vi "Main.vi"() -> ()   [LabVIEW 2020]
doc: "This template is for the Queued Message Handler design pattern.\n\nThe Event Handling Loop generates messages based on user interface actions.\n\nThe Message Handling Loop processes messages generated by the Event Handling Loop, or by other messages. The messages are string values, so new messages can be added easily to the Message Cases case structure in the Message Handling Loop. Each message cluster can also provide an optional value for Message Data, which is a variant that can be converted to whatever message-specific data is required."
uses:
  controls/Search button.ctl
  Panther Dashboard Library/Module type--enum.ctl
  controls/UI Data.ctl
  Panther Dashboard Library/DQMH Modules Info--cluster.ctl
  Panther Dashboard Library/Documentation--cluster.ctl
  support/User Event - Stop/User Events Refs--cluster.ctl
  Panther Dashboard Library/Project Name and Ref--cluster.ctl
  Panther Dashboard Library/Maps List and refs--cluster.ctl
  <vilib>/National Instruments/Tree Map/Tree Map Data.ctl
  <vilib>/Utility/miscctls.llb/LVPointTypeDef.ctl
  support/Message Queue/Enqueue Message (Array).vi
  support/Message Queue/Enqueue Message (Single).vi
  <vilib>/National Instruments/Tree Map/API/List Roots.vi
  <vilib>/National Instruments/Tree Map/Utility/Into Tree Control Items.vi
  <vilib>/Utility/error.llb/Error Cluster From Error Code.vi
  <vilib>/ErrorRing/Error Ring.xnode
  support/Message Queue/Message Queue.lvlib
  support/User Event - Stop/User Events.lvlib
  <vilib>/National Instruments/Tree Map/Tree Map.lvlib
  Panther Dashboard Library/Panther Dashboard.lvlib
  PantherSniffer/Source/Libraries/MQTT_Client/MQTT_Client.lvlib
panel:
  in  "Include Dependencies":bool
  in  "Projects":string(combo)
  in  "Refresh":T1
  in  "DQMH List":string(tree) caption="Tree 2"
  out "Event Connector Pane":picture
  in  "Open Event FP":bool
  in  "Module ID":i32 caption="Numeric" format="Module ID : %d"
  in  "Show Diagram":bool
  in  "Hide Panel":bool
  in  "Show Panel":bool
  in  "Stop Instance":bool
  in  "Stop Module":bool
  out "Running?":bool
  out "Module type":T2
  in  "Open API Tester":bool
  out "Module Description":string
  out "Event Description":string
  out "Messages":string
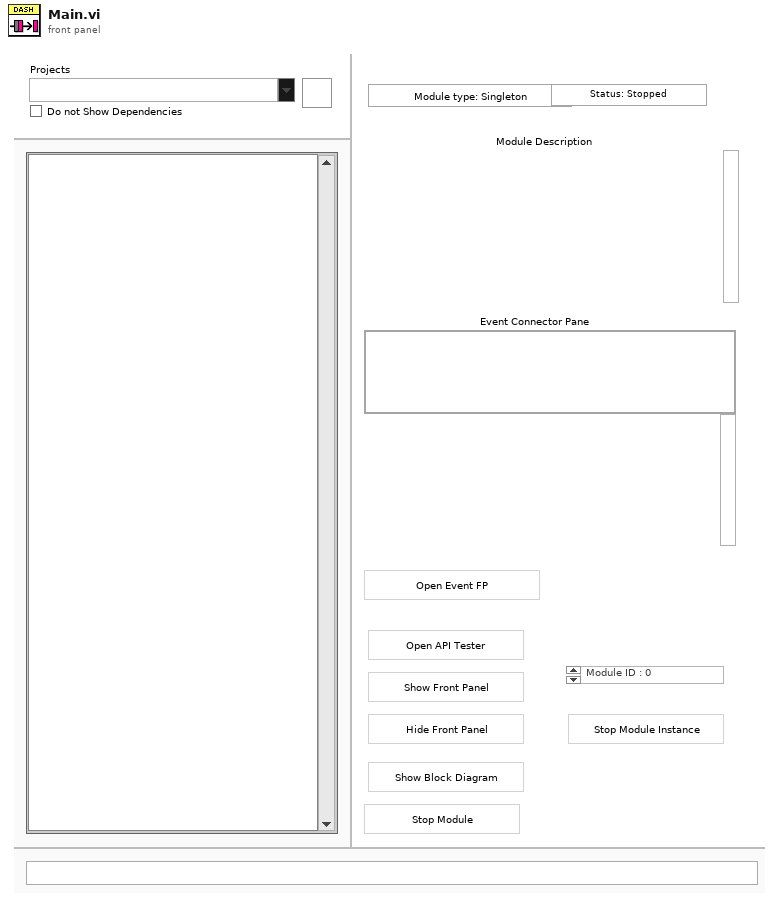
[diagram p1: front panel]
types:
  T1 = typedef "Search button.ctl" = bool
  T2 = typedef "Panther Dashboard.lvlib/Module type--enum.ctl" = enum16{"Module type: Singleton", "Module type: Cloneable"}
  T3 = typedef "UI Data.ctl" = cluster{"DQMH Modules Info":T4, "Documentation":T5, "FP Ctrs Refs":cluster{"Open API Tester":refnum<vi>, "Run Request VI":refnum<vi>, "Show Diagram":refnum<vi>, "Hide Panel":refnum<vi>, "Show Panel":refnum<vi>, "Stop All":refnum<vi>, "Stop Module":refnum<vi>}, "User Events":T6, "Project":T7, "UI Elements":cluster{"Connector pane img":picture, "Module selected type":T2, "DQMH Module Name":string, "Module ID":i32}, "DQMH Refs":cluster{"Event vi Ref":refnum<vi>, "DQMH Module Selected Ref":refnum<vi>}, "Maps":T8, "Tree Control Ref":refnum<vi>}
  T4 = typedef "Panther Dashboard.lvlib/DQMH Modules Info--cluster.ctl" = cluster{"DQMH Modules Refs":refnum<vi>[], "Modules List":string[], "Modules Descriptions":string[], "Modules Paths":path[], "Modules type":T2[]}
  T5 = typedef "Panther Dashboard.lvlib/Documentation--cluster.ctl" = cluster{"Module Description":string, "Event Description":string}
  T6 = typedef "User Events.lvlib/User Events Refs--cluster.ctl" = cluster{"Stop Event":refnum<user-event>, "Message event ":refnum<user-event>, "DQMH Mod Ref":refnum<user-event>}
  T7 = typedef "Panther Dashboard.lvlib/Project Name and Ref--cluster.ctl" = cluster{"Project Ref":refnum<vi>, "Project Name Selection":string, "Include Dependencies":bool}
  T8 = typedef "Panther Dashboard.lvlib/Maps List and refs--cluster.ctl" = cluster{"Tree Map":T9, "References Map":map{string, refnum<vi>}}
  T9 = typedef "Tree Map.lvlib/Tree Map Data.ctl" = map{string, cluster{"Child Paths Set":set{string}, "Name":string, "Data":string, "Attributes":map{string, string}}}
  T10 = typedef "Message Queue.lvlib/All Message Queues.ctl" = cluster{"UI":refnum<queue>}
  T11 = typedef "LVPointTypeDef.ctl" = cluster{"Horizontal":i16, "Vertical":i16}
  T12 = enum8{"Enabled", "Disabled", "Disabled and Grayed Out"}
  T13 = enum32{"Invalid", "Standard", "Closed", "Hidden", "Minimized", "Maximized"}
  T14 = cluster{"Open API Tester":refnum<vi>, "Open Event FP":refnum<vi>, "Show Diagram":refnum<vi>, "Hide Panel":refnum<vi>, "Show Panel":refnum<vi>, "Stop Instance":refnum<vi>, "Stop Module":refnum<vi>}
  T15 = cluster{"Left Cell String":string, "Child Text":string[], "Child Tag":string, "Item Indent":i32, "Child Only?":bool, "Glyph Index":i32}[]
  T16 = cluster{"Open API Tester":refnum<vi>, "Run Request VI":refnum<vi>, "Show Diagram":refnum<vi>, "Hide Panel":refnum<vi>, "Show Panel":refnum<vi>, "Stop All":refnum<vi>, "Stop Module":refnum<vi>}
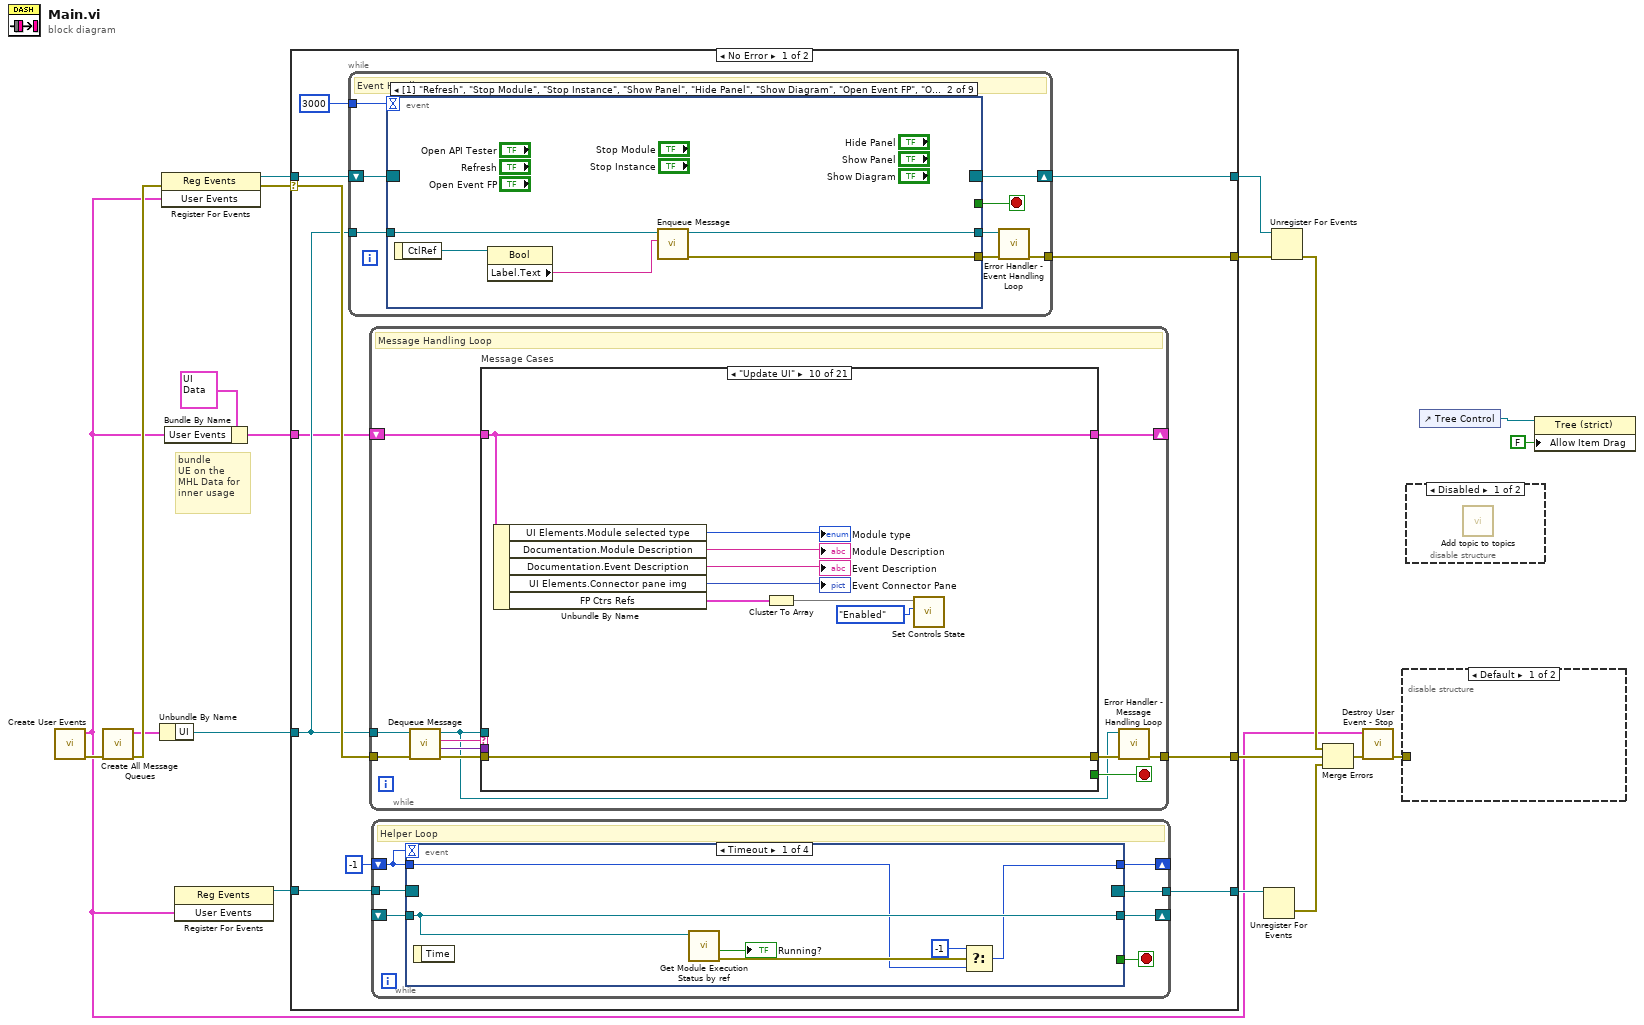
[diagram p0: block diagram]
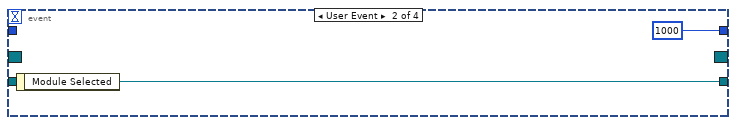
[diagram p3: hidden frame]
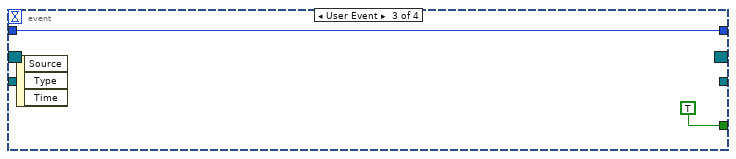
[diagram p4: hidden frame]
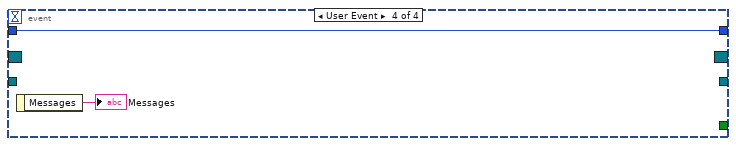
[diagram p5: hidden frame]
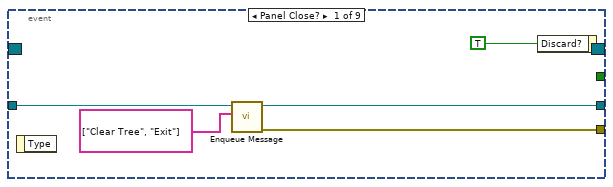
[diagram p6: hidden frame]
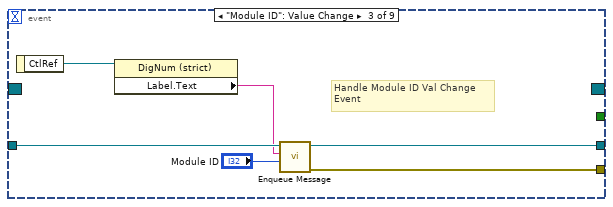
[diagram p7: hidden frame]
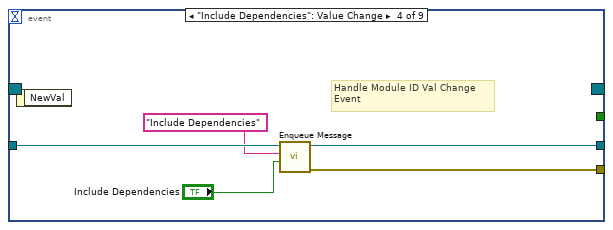
[diagram p8: hidden frame]
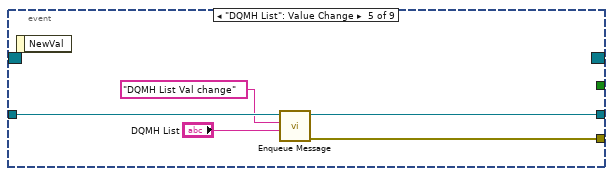
[diagram p9: hidden frame]
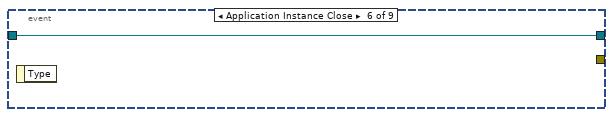
[diagram p10: hidden frame]
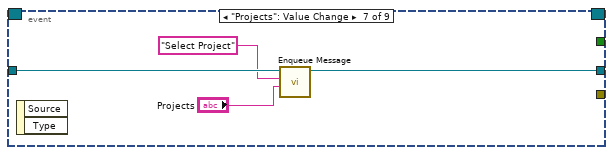
[diagram p11: hidden frame]
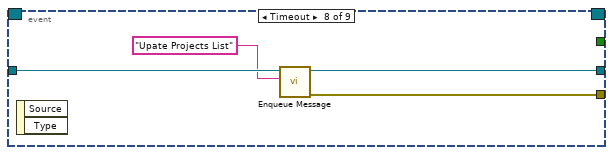
[diagram p12: hidden frame]
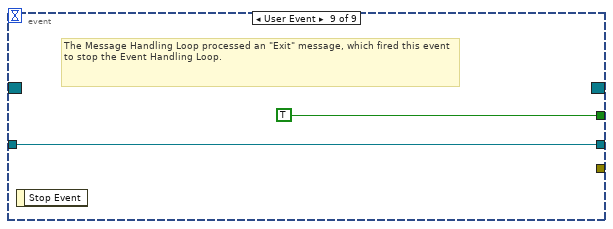
[diagram p13: hidden frame]
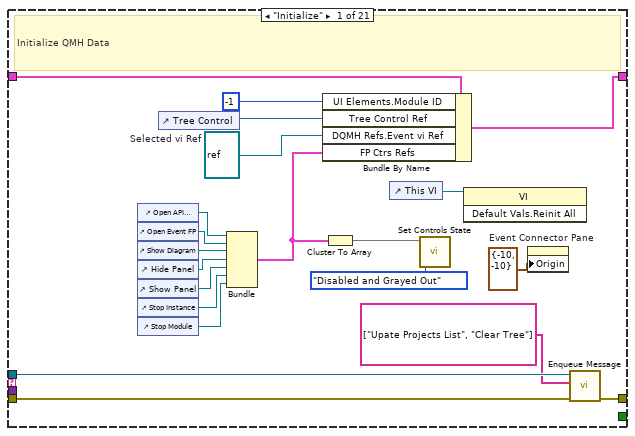
[diagram p14: hidden frame]
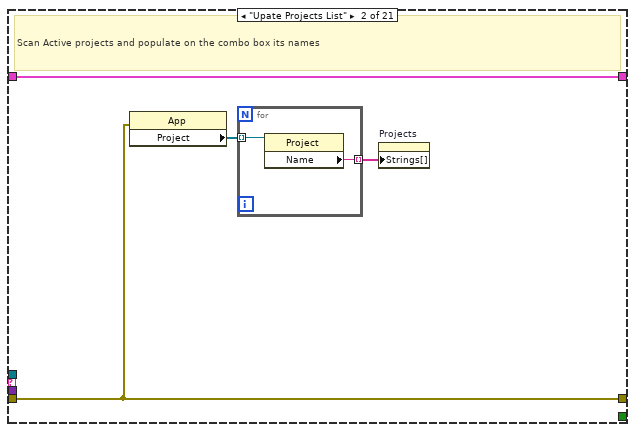
[diagram p15: hidden frame]
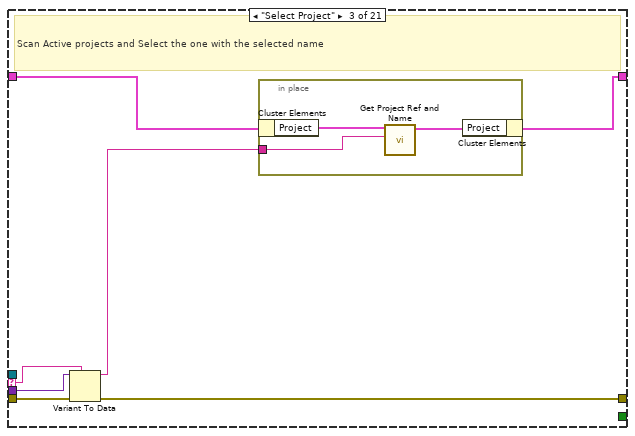
[diagram p16: hidden frame]
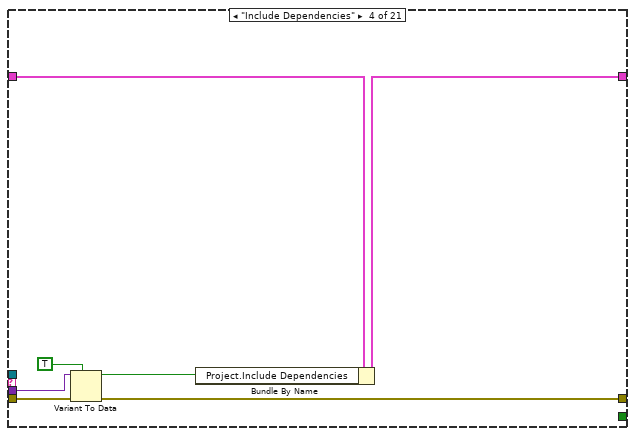
[diagram p17: hidden frame]
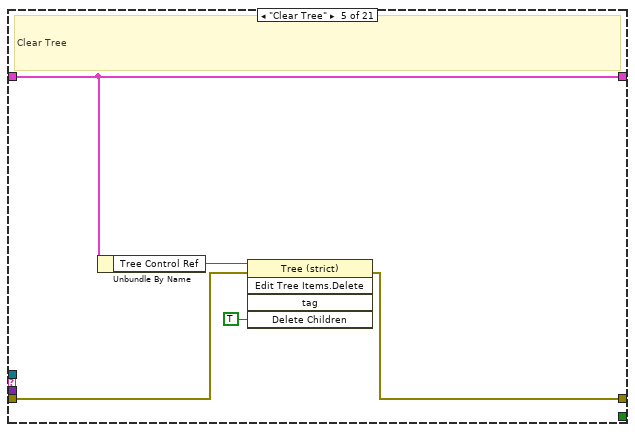
[diagram p18: hidden frame]
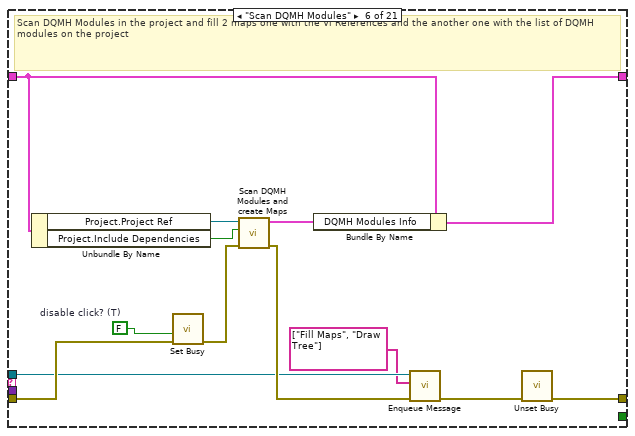
[diagram p19: hidden frame]
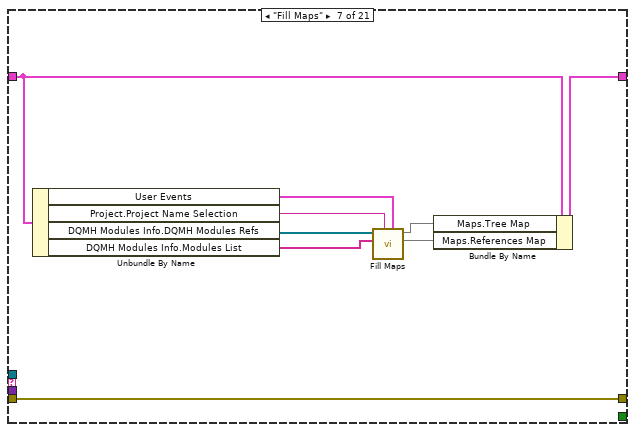
[diagram p20: hidden frame]
diagram:
  # "bundle\nUE on the\nMHL Data for\ninner usage"
  n1 = call "Create User Events.vi"() -> ("error out"=w19:errorcluster, "User Events"=w3:T6)  [unwired: 10 in]
  n2 = call "Create All Message Queues.vi"("error in (no error)"=w19) -> ("error out"=w13:errorcluster, "Message Queues out"=w11:T10)  [unwired: 9 in]
  n3 = Unbundle By Name(w11) -> ("UI"=w10:refnum<queue>)
  n4 = register-events(error in=w13, w3) -> (reference out=w7:refnum<event-registration>, error out=w12:errorcluster)  [unwired: 1 in]
  n5 = Bundle By Name(cluster=T3 {"DQMH Modules Info"={"DQMH Modules Refs"=[], "Modules List"=[], "Modules Descriptions"=[], "Modules Paths"=[], "Modules type"=[]}, "Documentation"={"Module Description"="", "Event Description"=""}, "FP Ctrs Refs"={"Open API Tester"=refnum, "Run Request VI"=refnum, "Show Diagram"=refnum, "Hide Panel"=refnum, "Show Panel"=refnum, "Stop All"=refnum, "Stop Module"=refnum}, "User Events"={"Stop Event"=refnum, "Message event "=refnum, "DQMH Mod Ref"=refnum}, "Project"={"Project Ref"=refnum, "Project Name Selection"="", "Include Dependencies"=FALSE}, "UI Elements"={"Connector pane img"=bytes[0], "Module selected type"=enum."Module type: Singleton", "DQMH Module Name"="", "Module ID"=0}, "DQMH Refs"={"Event vi Ref"=refnum, "DQMH Module Selected Ref"=refnum}, "Maps"={"Tree Map"={}, "References Map"={}}, "Tree Control Ref"=refnum} ("Data Cluster"), "User Events"=w3) -> (w6:T3)
  n6 = register-events(w3) -> (reference out=w5:refnum<event-registration>)  [unwired: 2 in, 1 out]
  n7 = case shown="No Error" w12 {
    selector: w12 -> [w29 w288]
    tunnel: [w31 _] -> w20
    tunnel: [w30 w288] -> w15
    tunnel: w10 -> [w28 _]
    tunnel: [w27 w287] -> w9
    tunnel: w7 -> [w26 w287]
    tunnel: w6 -> [w25 _]
    tunnel: w5 -> [w24 w286]
    tunnel: [w23 w286] -> w4
    frame No Error {
      n8 = while {
        tunnel: w28 -> [w56]
        shift-right: [w54] -> w27
        shift-left: w26 -> [w55]
        tunnel: [w57] -> w30
        tunnel: 3000 -> [w51]
        stop <- w53 stop-if-true
        # "Event Handling Loop"
        n9 = event shown="[1] \"Refresh\", \"Stop Module\", \"Stop Instance\", \"Show Panel\", \"Hide Panel\", \"Show Diagram\", \"Open Event FP\", \"Open API Tester\": Value Change" {
          selector: w55 -> [_ _ _ _ _ _ _ _ _]
          dyn-events: [_ _ _ _ _ _ _ _ _] -> w54
          timeout: w51 -> [_ _ _ _ _ _ _ _ _]
          tunnel: [_ _ _ _ _ _ _ _ TRUE ("Discard?")] -> w53
          tunnel: w56 -> [w61 w67 w73 w78 w84 w85 w89 w93 w95]
          tunnel: [w63 w68 w74 w79 w80 _ _ w90 _] -> w58
          tunnel: [w60 w65 w71 w77 w83 w85 w88 w92 w95] -> w52
          event Panel Close? {
            n10 = event-data() -> ()  [unwired: 1 in, 1 out]
            n11 = call-poly "Enqueue Message.vi"("Message Array"=string[] ["Clear Tree", "Exit"] ("Message"), "Message Queue"=w61) -> ("error out"=w63:errorcluster, "dup Message Queue"=w60:refnum<queue>)  [unwired: 8 in]
            n12 = event-data("Discard?"=TRUE) -> ()  [unwired: 1 in, 1 out]
          }
          event "Stop Module", "Stop Instance", "Show Panel", "Hide Panel", "Show Diagram", "Open Event FP", "Open API Tester": Value Change {
            n13 = event-data() -> ("CtlRef"=w66:refnum<vi>)  [unwired: 1 in]
            n14 = property class="Bool"(reference=w66) -> ("Label.Text"=w64:string)  [unwired: 1 in, 2 out]
            n15 = call-poly "Enqueue Message.vi"("Message"=w64, "Message Queue"=w67) -> ("error out"=w68:errorcluster, "dup Message Queue"=w65:refnum<queue>)  [unwired: 8 in]
          }
          event "Module ID": Value Change {
            # "Handle Module ID Val Change\nEvent"
            n16 = event-data() -> ("CtlRef"=w72:refnum<vi>)  [unwired: 1 in]
            n17 = property class="DigNum (strict)"(reference=w72) -> ("Label.Text"=w70:string)  [unwired: 1 in, 2 out]
            n18 = call-poly "Enqueue Message.vi"("Message Data"="Module ID", "Message"=w70, "Message Queue"=w73) -> ("error out"=w74:errorcluster, "dup Message Queue"=w71:refnum<queue>)  [unwired: 7 in]
          }
          event "Include Dependencies": Value Change {
            # "Handle Module ID Val Change\nEvent"
            n19 = event-data() -> ()  [unwired: 1 in, 1 out]
            n20 = call-poly "Enqueue Message.vi"("Message Data"="Include Dependencies", "Message"="Include Dependencies", "Message Queue"=w78) -> ("error out"=w79:errorcluster, "dup Message Queue"=w77:refnum<queue>)  [unwired: 7 in]
          }
          event "DQMH List": Value Change {
            n21 = event-data() -> ()  [unwired: 1 in, 1 out]
            n22 = call-poly "Enqueue Message.vi"("Message Data"="DQMH List", "Message"="DQMH List Val change", "Message Queue"=w84) -> ("error out"=w80:errorcluster, "dup Message Queue"=w83:refnum<queue>)  [unwired: 7 in]
          }
          event Application Instance Close {
            n23 = event-data() -> ()  [unwired: 1 in, 1 out]
          }
          event "Projects": Value Change {
            n24 = event-data() -> ()  [unwired: 1 in, 2 out]
            n25 = call-poly "Enqueue Message.vi"("Message Data"="Projects", "Message"="Select Project", "Message Queue"=w89) -> ("dup Message Queue"=w88:refnum<queue>)  [unwired: 7 in, 1 out]
          }
          event Timeout {
            n26 = event-data() -> ()  [unwired: 1 in, 2 out]
            n27 = call-poly "Enqueue Message.vi"("Message"="Upate Projects List", "Message Queue"=w93) -> ("error out"=w90:errorcluster, "dup Message Queue"=w92:refnum<queue>)  [unwired: 8 in]
          }
          event User Event {
            # "The Message Handling Loop processed an \"Exit\" message, which fired this event to stop the Event Handling Loop."
            n28 = event-data() -> ()  [unwired: 1 in, 1 out]
          }
        }
        n29 = call "Error Handler - Event Handling Loop.vi"("error in (no error)"=w58, "Message Queue"=w52) -> ("dup error in"=w57:errorcluster)  [unwired: 8 in, 1 out]
      }
      n30 = while {
        tunnel: w28 -> [w97]
        shift-right: [w101] -> _
        shift-left: w25 -> [w102]
        tunnel: w29 -> [w106]
        tunnel: [w104] -> w31
        stop <- w100 stop-if-true
        # "Message Handling Loop"
        n31 = call "Dequeue Message.vi"("error in (no error)"=w106, "Message Queue"=w97) -> ("error out"=w105:errorcluster, "Message Data"=w98:variant, "Message"=w99:string, "dup Message Queue"=w96:refnum<queue>)  [unwired: 6 in]
        n32 = case "Message Cases" shown="\"Update UI\"" w99 {
          selector: w99 -> [_ _ w137 _ _ _ _ _ _ _ _ w217 _ _ _ _ _ _ _ _ w276]
          tunnel: w96 -> [w123 _ _ _ _ w161 _ _ w192 _ _ _ _ w231 _ _ _ _ _ w269 _]
          tunnel: w105 -> [w127 w128 w140 w150 w155 w167 w177 w184 w203 w212 _ w223 w229 w235 w240 w246 w253 w260 w263 w272 _]
          tunnel: [w126 w128 w139 w148 w154 w164 w177 w183 w201 w212 w213 w222 w228 w234 w239 w245 w252 w256 w262 w274 w278] -> w103
          tunnel: w102 -> [w125 w131 w136 w149 w152 w160 w176 w181 w198 w211 w216 w220 w225 w233 w237 w244 w251 w255 w261 w266 w277]
          tunnel: [w124 w131 w134 w145 w152 w163 w172 w181 w196 w211 w216 w220 w225 w233 w237 w244 w248 w255 w261 w266 w277] -> w101
          tunnel: [_ _ _ _ _ _ _ _ _ _ _ _ _ _ _ _ _ _ _ TRUE _] -> w100
          tunnel: w98 -> [_ _ w138 w147 _ _ _ _ w200 _ _ _ _ _ _ _ w250 w254 _ w267 _]
          frame "Initialize" {
            w107 = refnum<vi> refnum  # Selected vi Ref
            # "Initialize QMH Data"
            n33 = control-ref of="Open API Tester"() -> (w115:refnum<vi>)
            n34 = control-ref of="Open Event FP"() -> (w116:refnum<vi>)
            n35 = control-ref of="Show Diagram"() -> (w117:refnum<vi>)
            n36 = control-ref of="Hide Panel"() -> (w118:refnum<vi>)
            n37 = control-ref of="Show Panel"() -> (w119:refnum<vi>)
            n38 = control-ref of="Stop Instance"() -> (w120:refnum<vi>)
            n39 = control-ref of="Stop Module"() -> (w121:refnum<vi>)
            n40 = control-ref of="Tree Control"() -> (w108:refnum<vi>)
            n41 = Bundle("Open API Tester"=w115, "Open Event FP"=w116, "Show Diagram"=w117, "Hide Panel"=w118, "Show Panel"=w119, "Stop Instance"=w120, "Stop Module"=w121) -> (w110:T14)  [unwired: 1 in]
            n42 = Bundle By Name(cluster=w125, "UI Elements.Module ID"=-1 ("Module ID"), "Tree Control Ref"=w108, "DQMH Refs.Event vi Ref"=w107, "FP Ctrs Refs"=w110) -> (w124:T3)
            n43 = Cluster To Array(cluster=w110) -> (array=w114:refnum<vi>[])
            n44 = control-ref of="This VI"() -> (w112:refnum<vi>)
            n45 = call "Set Controls State.vi"("Disabled"=T12."Disabled and Grayed Out", "Ctrl Refs"=w114) -> ()  [unwired: 10 in]
            n46 = invoke class="VI" method="Default Vals.Reinit All"(reference=w112) -> ()  [unwired: 2 in, 3 out]
            n47 = property on="Event Connector Pane" class="Pict"("Origin"=T11 {"Horizontal"=-10, "Vertical"=-10}) -> ()  [unwired: 2 in, 2 out]
            n48 = call-poly "Enqueue Message.vi"("error in (no error)"=w127, "Message Array"=string[] ["Upate Projects List", "Clear Tree"] ("Initial Step"), "Message Queue"=w123) -> ("error out"=w126:errorcluster)  [unwired: 7 in, 1 out]
          }
          frame "Upate Projects List" {
            # "Scan Active projects and populate on the combo box its names"
            n49 = property class="App"(error in=w128) -> ("Project"=w130:refnum<vi>[])  [unwired: 1 in, 2 out]
            n50 = for {
              tunnel: w130 -> [w133] mode=indexing
              tunnel: [w132] -> w129 mode=indexing
              n51 = property class="Project"(reference=w133) -> ("Name"=w132:string)  [unwired: 1 in, 2 out]
            }
            n52 = property on="Projects" class="CmbBox"("Strings[]"=w129) -> ()  [unwired: 2 in, 2 out]
          }
          frame "Select Project" {
            # "Scan Active projects and Select the one with the selected name"
            n53 = Variant To Data(error in=w140, type=w137, Variant=w138) -> (data=w135:string, error out=w139:errorcluster)
            n54 = in-place {
              in-place-border: w135 -> [w143]
              n55 = in-place-cluster #1(w136) -> ("Project"=w141:T7)
              n56 = call "Get Project Ref and Name.vi"("Project Name Selection"=w143, "ProjectIn"=w141) -> ("Project out"=w142:T7)  [unwired: 9 in]
              n57 = in-place-cluster #1("Project"=w142) -> (w134:T3)
            }
          }
          frame "Include Dependencies" {
            n58 = Variant To Data(error in=w150, type=TRUE, Variant=w147) -> (data=w144:bool, error out=w148:errorcluster)
            n59 = Bundle By Name(cluster=w149, "Project.Include Dependencies"=w144) -> (w145:T3)
          }
          frame "Clear Tree" {
            # "Clear Tree"
            n60 = Unbundle By Name(w152) -> ("Tree Control Ref"=w151:refnum<vi>)
            n61 = invoke on="Invoke Node" class="Tree (strict)" method="Edit Tree Items.Delete"(reference=w151, error in=w155, "Delete Children"=TRUE ("Delete Children?")) -> (error out=w154:errorcluster)  [unwired: 2 in, 4 out]
          }
          frame "Scan DQMH Modules" {
            w158 = FALSE  # disable click? (T)
            # "Scan DQMH Modules in the project and fill 2 maps one with the Vi References and the another one with the list of DQMH modules on the project"
            n62 = Unbundle By Name(w160) -> ("Project.Project Ref"=w159:refnum<vi>, "Project.Include Dependencies"=w156:bool)
            n63 = call <vilib>:"Set Busy.vi"("error in (no error)"=w167, "disable click? (T)"=w158) -> ("error out"=w166:errorcluster)  [unwired: 8 in, 1 out]
            n64 = call "Scan DQMH Modules and create Maps.vi"("error in"=w166, "Include Dependencies"=w156, "Project"=w159) -> ("error out"=w168:errorcluster, "DQMH Modules Info"=w162:T4)  [unwired: 7 in]
            n65 = Bundle By Name(cluster=w160, "DQMH Modules Info"=w162) -> (w163:T3)
            n66 = call-poly "Enqueue Message.vi"("error in (no error)"=w168, "Message Array"=string[] ["Fill Maps", "Draw Tree"] ("Message"), "Message Queue"=w161) -> ("error out"=w165:errorcluster)  [unwired: 7 in, 1 out]
            n67 = call <vilib>:"Unset Busy.vi"("error in (no error)"=w165) -> ("error out"=w164:errorcluster)  [unwired: 10 in]
          }
          frame "Fill Maps" {
            n68 = Unbundle By Name(w176) -> ("User Events"=w169:T6, "Project.Project Name Selection"=w173:string, "DQMH Modules Info.DQMH Modules Refs"=w175:refnum<vi>[], "DQMH Modules Info.Modules List"=w174:string[])
            n69 = call "Fill Maps.vi"("User Events"=w169, "Project Selected"=w173, "Module names"=w174, "DQMH Modules"=w175) -> ("map ref out"=w170:map{string, refnum<vi>}, "Tree Map out"=w171:T9)  [unwired: 5 in, 1 out]
            n70 = Bundle By Name(cluster=w176, "Maps.Tree Map"=w171, "Maps.References Map"=w170) -> (w172:T3)
          }
          frame "Draw Tree" {
            # "Draw  DQMH List with all the DQMH Modules listed, first we need to clean the tree list"
            n71 = Unbundle By Name(w181) -> ("Tree Control Ref"=w178:refnum<vi>, "Maps.Tree Map"=w180:T9)
            n72 = call <vilib>:"Tree Map to Tree Control Items.vi"("Tree Map In"=w180) -> ("Tree Control Items"=w179:T15)  [unwired: 10 in]
            n73 = call "Draw Tree.vi"("Tree Control Items"=w179, "TreeControl in"=w178) -> ("error out"=w182:errorcluster)  [unwired: 9 in]
            n74 = Merge Errors(w182, w184) -> (w183:errorcluster)
          }
          frame "DQMH List Val change" {
            # "DQMH List has a value change"
            n75 = Unbundle By Name(w198) -> ("Maps.Tree Map"=w197:T9, "Maps.References Map"=w194:map{string, refnum<vi>}, "DQMH Modules Info"=w193:T4)
            n76 = Variant To Data(error in=w203, type="" ("DQMH List"), Variant=w200) -> (data=w195:string, error out=w202:errorcluster)
            n77 = call "Get List Information.vi"("List Selection"=w195, "DQMH Modules Info"=w193, "References Map"=w194, "Tree Map"=w197) -> ("Documentation"=w190:T5, "Module Type"=w188:T2, "Vi out"=w187:refnum<vi>, "Library name"=w186:string, "VI Connector Pane"=w189:picture, "DQMH Lib"=w185:refnum<vi>)  [unwired: 2 in]
            n78 = Bundle By Name(cluster=w198, "DQMH Refs.DQMH Module Selected Ref"=w185, "UI Elements.DQMH Module Name"=w186, "DQMH Refs.Event vi Ref"=w187, "UI Elements.Module selected type"=w188, "Documentation"=w190, "UI Elements.Connector pane img"=w189) -> (w196:T3)
            n79 = call-poly "Enqueue Message.vi"("error in (no error)"=w202, "Message Array"=string[] ["Get Module Status", "Update UI"] ("Message"), "Message Queue"=w192) -> ("error out"=w201:errorcluster)  [unwired: 7 in, 1 out]
          }
          frame "Update UI" {
            n80 = Unbundle By Name(w211) -> ("UI Elements.Module selected type"=→"Module type":T2, "Documentation.Module Description"=→"Module Description":string, "Documentation.Event Description"=→"Event Description":string, "UI Elements.Connector pane img"=→"Event Connector Pane":picture, "FP Ctrs Refs"=w205:T16)
            n81 = Cluster To Array(cluster=w205) -> (array=w204:refnum<vi>[])
            n82 = call "Set Controls State.vi"("Disabled"=T12."Enabled", "Ctrl Refs"=w204) -> ()  [unwired: 10 in]
          }
          frame "Get Module Status" {
            n83 = Unbundle By Name(w216) -> ("User Events.DQMH Mod Ref"=w215:refnum<user-event>, "DQMH Refs.DQMH Module Selected Ref"=w214:refnum<vi>)
            n84 = Generate User Event(user event=w215, event data cluster=w214) -> (error out=w213:errorcluster)  [unwired: 2 in, 1 out]
          }
          frame "Hide Panel", "Show Diagram", "Show Panel", "Stop Module" {
            # "Search for the vi ref of the selected events {Hide Panel, Show Diagram, Show Panel,\"Stop Module\"}"
            n85 = Unbundle By Name(w220) -> ("Maps.References Map"=w219:map{string, refnum<vi>}, "UI Elements.DQMH Module Name"=w218:string)
            n86 = call "Find and trigger default events.vi"("Event to Trigger"=w217, "Library Selected"=w218, "References Map"=w219) -> ("error out"=w221:errorcluster)  [unwired: 8 in]
            n87 = Merge Errors(w221, w223) -> (w222:errorcluster)
          }
          frame "Stop Instance" {
            n88 = Unbundle By Name(w225) -> ("Maps.References Map"=w227:map{string, refnum<vi>}, "UI Elements.DQMH Module Name"=w226:string, "UI Elements.Module ID"=w224:i32)
            n89 = call "Stop by ID.vi"("Module ID"=w224, "Library Selected"=w226, "References Map"=w227) -> ("error out"=w230:errorcluster)  [unwired: 8 in]
            n90 = Merge Errors(w230, w229) -> (w228:errorcluster)
          }
          frame "Refresh" {
            # "Refresh the projects available"
            n91 = call-poly "Enqueue Message.vi"("error in (no error)"=w235, "Message"="Scan DQMH Modules" ("Steps"), "Message Queue"=w231) -> ("error out"=w234:errorcluster)  [unwired: 7 in, 1 out]
          }
          frame "Open API Tester" {
            n92 = Unbundle By Name(w237) -> ("DQMH Refs.DQMH Module Selected Ref"=w236:refnum<vi>)
            n93 = call "Open API Tester.vi"("DQMH Library Ref"=w236) -> ("error out"=w238:errorcluster)  [unwired: 10 in]
            n94 = Merge Errors(w238, w240) -> (w239:errorcluster)
          }
          frame "Open Event FP" {
            n95 = Unbundle By Name(w244) -> ("DQMH Refs.Event vi Ref"=w243:refnum<vi>)
            n96 = invoke class="VI" method="FP.Open"(reference=w243, error in=w246, "Activate"=TRUE ("Wait Until Done"), "State"=T13."Standard") -> (error out=w245:errorcluster)  [unwired: 1 in, 4 out]
          }
          frame "Module ID" {
            # "Module ID changed"
            n97 = Variant To Data(error in=w253, type=0 ("Module ID"), Variant=w250) -> (data=w247:i32, error out=w252:errorcluster)
            n98 = Bundle By Name(cluster=w251, "UI Elements.Module ID"=w247) -> (w248:T3)
          }
          frame "Error" {
            # "Error - Display an error dialog. This message is sent by the \"Error Handler\" VIs at the end of other loops in this application."
            n99 = Variant To Data(error in=w260, type=errorcluster {"status"=FALSE, "code"=0, "source"=""} ("error constant"), Variant=w254) -> (data=w258:errorcluster, error out=w257:errorcluster)
            n100 = call <vilib>:"Simple Error Handler.vi"("error in (no error)"=w258) -> ()  [unwired: 4 in, 5 out]
            n101 = Merge Errors(w257) -> (w256:errorcluster)
          }
          frame "---Copy This Frame---" {
            # "Duplicate this frame when creating new messages.  Change this comment in the duplicated frame to describe this message."
            n102 = Merge Errors(w263) -> (w262:errorcluster)
          }
          frame "Exit" {
            # "Stop the VI"
            # "Release the message queue reference"
            # "Exit - Exit the application."
            n103 = Variant To Data(type=errorcluster {"status"=FALSE, "code"=0, "source"=""} ("error constant"), Variant=w267) -> (data=w270:errorcluster)  [unwired: 1 in, 1 out]
            n104 = call <vilib>:"Simple Error Handler.vi"("error in (no error)"=w270) -> ()  [unwired: 4 in, 5 out]
            n105 = Unbundle By Name(w266) -> ("Maps.References Map"=w265:map{string, refnum<vi>}, "User Events.Stop Event"=w264:refnum<user-event>)
            n106 = Release Queue(queue=w269, error in (no error)=w272) -> (error out=w275:errorcluster)  [unwired: 1 in, 2 out]
            n107 = call "Fire User Event - Stop.vi"("User Event - Stop"=w264) -> ("error out"=w273:errorcluster)  [unwired: 10 in]
            n108 = call "Close vi references.vi"("map"=w265) -> ()  [unwired: 11 in]
            n109 = Merge Errors(w273, w275) -> (w274:errorcluster)
          }
          frame Default {
            # "'Default' case only runs if there is a message that isn't defined in any of the other cases.  Output a programming error."
            n110 = xnode "Error Ring"("parameter 0"=w276) -> ("error out"=w278:errorcluster)
          }
        }
        n111 = call "Error Handler - Message Handling Loop.vi"("error in (no error)"=w103, "Message Queue"=w96) -> ("dup error in"=w104:errorcluster)  [unwired: 8 in, 1 out]
      }
      n112 = while {
        tunnel: w24 -> [w38]
        tunnel: [w37] -> w23
        shift-right: [w35] -> _
        shift-left: _ -> [w34]
        shift-right: [w33] -> _
        shift-left: -1 -> [w32]
        stop <- w36 stop-if-true
        # "Helper Loop"
        n113 = event shown="[0] Timeout" {
          selector: w38 -> [_ _ _ _]
          dyn-events: [_ _ _ _] -> w37
          timeout: w32 -> [_ _ _ _]
          tunnel: [_ _ TRUE _] -> w36
          tunnel: [w43 w46 _ _] -> w35
          tunnel: w34 -> [w43 _ _ _]
          tunnel: [w39 1000 w47 w49] -> w33
          tunnel: w32 -> [w41 _ w47 w49]
          event Timeout {
            n114 = event-data() -> ()  [unwired: 1 in, 1 out]
            n115 = call "Get Module Execution Status by ref.vi"("Library"=w43) -> ("error out"=w42:errorcluster, "Running?"=→"Running?":bool)  [unwired: 8 in, 1 out]
            n116 = Select(t=-1, s=w42, f=w41) -> (s? t:f=w39:i32)
          }
          event User Event {
            n117 = event-data() -> ("Module Selected"=w46:refnum<vi>)  [unwired: 1 in]
          }
          event User Event {
            n118 = event-data() -> ()  [unwired: 1 in, 3 out]
          }
          event User Event {
            n119 = event-data() -> ("Messages"=→"Messages":string)  [unwired: 1 in]
          }
        }
      }
    }
    frame Error {
    }
  }
  n120 = Unregister For Events(event registration refnum=w4) -> (error out=w14:errorcluster)  [unwired: 1 in]
  n121 = Unregister For Events(event registration refnum=w9, error in=w15) -> (error out=w17:errorcluster)
  n122 = Merge Errors(w17, w20, w14) -> (w18:errorcluster)
  n123 = call "Destroy User Event - Stop.vi"("error in"=w18, "User Events"=w3) -> ("error out"=w16:errorcluster)  [unwired: 9 in]
  n124 = disable-structure shown="Default" {
    disable-tunnel: w16 -> [_ _]
    frame condition #0 (active) {
    }
    frame condition #1 {
      # "Call Quit LabVIEW if running as a built application."
      n125 = Quit LabVIEW() -> ()  [unwired: 1 in]
    }
  }
  n126 = disable-structure shown="Disabled" {
    frame Disabled {
      n127 = call "Add topic to topics.vi"() -> ()  [unwired: 11 in, 1 out]
    }
    frame Enabled {
    }
  }
  n128 = control-ref of="Tree Control"() -> (w2:refnum<vi>)
  n129 = property class="Tree (strict)"(reference=w2, "Allow Item Drag"=FALSE ("Drag/Drop:Allow Dragging")) -> ()  [unwired: 1 in, 2 out]
